vi "PH_Img_BaseClass.set Palette.vi"(0 "i ref in":refnum<vi>, 2 "Palette":T1 items=["Grey", "Binary", "Gradient", "Rainbow", "Temperature"], 5 "error in (no error)":errorcluster) -> (14 "i ref out":refnum<vi>, 19 "error out":errorcluster)   [LabVIEW 2014, in "PH_Img_BaseClass.lvlib"]
uses:
  PH_Img_BaseClass.lvlib
  PH_Img_BaseClass.Palette.ctl
  PH_Common/PH_Common.lvlib
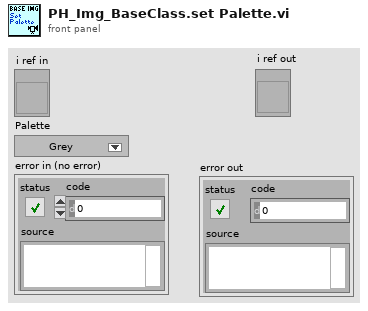
[diagram p1: front panel]
types:
  T1 = typedef "PH_Img_BaseClass.lvlib/PH_Img_BaseClass.Palette.ctl" = i32
  T2 = typedef "PH_Img_BaseClass.lvlib/PH_Img_BaseClass.i attribute.ctl" = cluster{"GUI Refs":T3, "Timeout Image [ms]":i32, "Default Periodic Period [ms]":i32, "Camera":cluster{"Instancename":string, "Notifier":refnum<notifier>}, "Palette":T1, "Cam Settings":cluster{"Cam ID":string, "Gain":dbl, "Brightness":dbl, "Shutter":dbl, "Cam Info Failure":bool, "Mode":i32}}
  T3 = typedef "PH_Img_BaseClass.lvlib/PH_Img_BaseClass.GUI Refs.ctl" = cluster{"Timeout":refnum<vi>, "Image":refnum<vi>, "Palette":refnum<vi>, "Timeout Set":refnum<vi>}
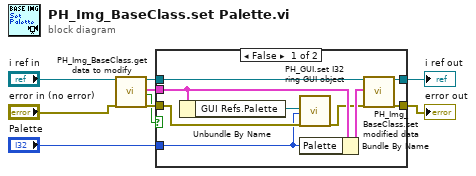
[diagram p0: block diagram]
diagram:
  n1 = call "PH_Img_BaseClass.get data to modify.vi"("i ref in"="i ref in", "error in (no error)"="error in (no error)") -> ("i ref out"=w9:refnum<vi>, "i attribute"=w3:T2, "timed out"=w2:bool, "error out"=w6:errorcluster)  [unwired: 14 in]
  n2 = case shown="False" w2 {
    tunnel: w9 -> [w18 w20]
    tunnel: [w17 w19] -> w7
    tunnel: w6 -> [w16 w19]
    tunnel: [w15 w20] -> w4
    tunnel: w3 -> [w13 _]
    tunnel: "Palette" -> [w10 _]
    frame False {
      n3 = Unbundle By Name(w13) -> ("GUI Refs.Palette"=w11:refnum<vi>)
      n4 = call "PH_GUI.set I32 ring GUI object.vi"("Ring Ref"=w11, "Value"=w10, "error in (no error)"=w16) -> ("error out"=w12:errorcluster)  [unwired: 16 in]
      n5 = Bundle By Name(cluster=w13, "Palette"=w10) -> (w14:T2)
      n6 = call "PH_Img_BaseClass.set modified data.vi"("i ref in"=w18, "i attribute"=w14, "error in (no error)"=w12) -> ("i ref out"=w15:refnum<vi>, "error out"=w17:errorcluster)  [unwired: 15 in]
    }
    frame True {
    }
  }
  "error out" <- w7
  "i ref out" <- w4
